vi "TCPROSSubscriberInit.vi"(2 "topic":string, 3 "callerID":string) -> (1 "TCP ROS Reply":string)   [LabVIEW 2015]
uses:
  MessageBuilding/std_msgs/subs/stringArray.vi
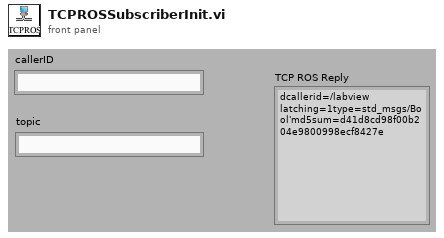
[diagram p1: front panel]
types:
  T1 = typedef "_ROSControl.ctl" = cluster{"topic port":u16, "Node":string, "topic":string, "type":string, "node port":u32, "error ":errorcluster, "Direction":T2, "APIs":string[]}
  T2 = typedef "_ROSDirection.ctl" = enum16{"Node", "Publisher", "Subscriber", "Service Client"}
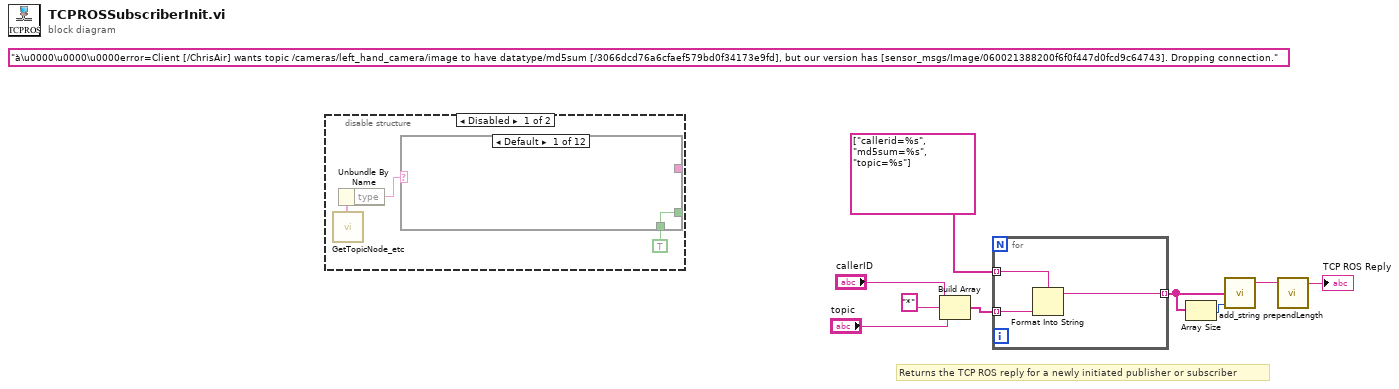
[diagram p0: block diagram]
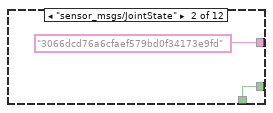
[diagram p2: hidden frame]
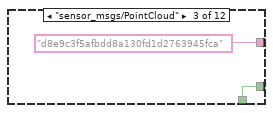
[diagram p3: hidden frame]
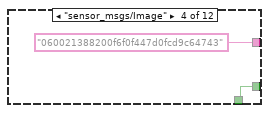
[diagram p4: hidden frame]
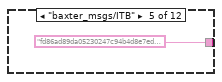
[diagram p5: hidden frame]
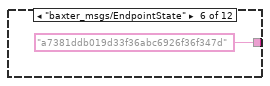
[diagram p6: hidden frame]
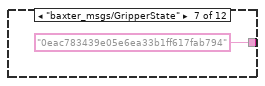
[diagram p7: hidden frame]
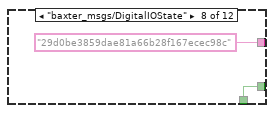
[diagram p8: hidden frame]
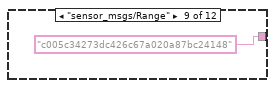
[diagram p9: hidden frame]
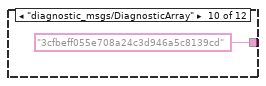
[diagram p10: hidden frame]
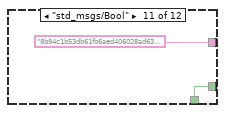
[diagram p11: hidden frame]
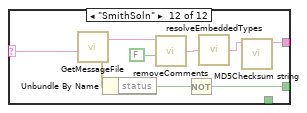
[diagram p12: hidden frame]
diagram:
  (unwired) "à\u0000\u0000\u0000error=Client [/ChrisAir] wants topic /cameras/left_hand_camera/image to have datatype/md5sum [/3066dcd76a6cfaef579bd0f34173e9fd], but our version has [sensor_msgs/Image/060021388200f6f0f447d0fcd9c64743]. Dropping connection." ("Second")
  # "Returns the TCP ROS reply for a newly initiated publisher or subscriber"
  n1 = disable-structure shown="Disabled" {
    frame Disabled {
      n2 = call "GetTopicNode_etc.vi"() -> ("ROS"=w12:T1)  [unwired: 3 in]
      n3 = Unbundle By Name(w12) -> ("type"=w10:string)
      n4 = case shown="Default" w10 {
        selector: w10 -> [_ _ _ _ _ _ _ _ _ _ _ w33]
        tunnel: [_ "3066dcd76a6cfaef579bd0f34173e9fd" "d8e9c3f5afbdd8a130fd1d2763945fca" "060021388200f6f0f447d0fcd9c64743" ("MD5 Sum") "fd86ad89da05230247c94b4d8e7ed306" ("MD5 Sum") "a7381ddb019d33f36abc6926f36f347d" ("MD5 Sum") "0eac783439e05e6ea33b1ff617fab794" ("MD5 Sum") "29d0be3859dae81a66b28f167ecec98c" ("MD5 Sum") "c005c34273dc426c67a020a87bc24148" ("Second") "3cfbeff055e708a24c3d946a5c8139cd" ("MD5 Sum") "8b94c1b53db61fb6aed406028ad6332a" ("MD5 Sum") w29] -> _
        tunnel: [w13 w14 w16 w18 _ _ _ w23 _ _ w27 w31] -> _
        tunnel: TRUE ("status") -> [w13 w14 w16 w18 _ _ _ w23 _ _ w27 _]
        frame Default {
        }
        frame "sensor_msgs/JointState" {
        }
        frame "sensor_msgs/PointCloud" {
        }
        frame "sensor_msgs/Image" {
        }
        frame "baxter_msgs/ITB" {
        }
        frame "baxter_msgs/EndpointState" {
        }
        frame "baxter_msgs/GripperState" {
        }
        frame "baxter_msgs/DigitalIOState" {
        }
        frame "sensor_msgs/Range" {
        }
        frame "diagnostic_msgs/DiagnosticArray" {
        }
        frame "std_msgs/Bool" {
        }
        frame "SmithSoln" {
          n5 = call "GetMessageFile.vi"("type"=w33) -> ("error out"=w34:errorcluster, "File"=w35:string)  [unwired: 1 in]
          n6 = Unbundle By Name(w34) -> ("status"=w32:bool)
          n7 = call "removeComments.vi"("Trim Whitespace? (F)"=FALSE ("Trim Whitespace?"), "String"=w35) -> ("Body"=w37:string)  [unwired: 2 in, 2 out]
          n8 = Not(x=w32) -> (.not. x?=w31:bool)
          n9 = call "resolveEmbeddedTypes.vi"("Message Definition"=w37) -> ("Md5 Text"=w30:string)
          n10 = call "MD5Checksum string.vi"("Message String"=w30) -> ("MD5 message-digest"=w29:string)  [unwired: 10 in]
        }
      }
    }
    frame Enabled {
    }
  }
  n11 = Build Array("callerID", "*", "topic") -> (w8:string[])
  n12 = for {
    tunnel: w8 -> [w39] mode=indexing
    tunnel: string[] ["callerid=%s", "md5sum=%s", "topic=%s"] -> [w40] mode=indexing
    tunnel: [w38] -> w1 mode=indexing
    n13 = Format Into String(format string=w40, w39) -> (resulting string=w38:string)  [unwired: 2 in, 1 out]
  }
  n14 = Array Size(array=w1) -> (size(s)=w2:i32)
  n15 = call-poly "add_string.vi"("Array Length"=w2, "Array"=w1) -> ("msg out"=w5:string)  [unwired: 3 in]
  n16 = call "prependLength.vi"("msg in"=w5) -> ("msg out"=→"TCP ROS Reply":string)  [unwired: 4 in]
